vi "Runtime Test.vi"() -> ()   [LabVIEW 2015, in "Numeric Limit Compare Tests.lvlib"]
uses:
  Numeric Limit Compare Tests.lvlib
  Config/Numeric Limit Compare Config.lvclass
  <vilib>/NI/Tag Bus/tag/Data Type.ctl
  <vilib>/NI/Tag Bus Module Framework/channel/channel classification.ctl
  classes/Step/Execution/StepState.ctl
  classes/Step/Execution/Step State Enum.ctl
  classes/Step/Execution/Step Flow Control.ctl
  Config/Comparison Types.ctl
  Config/Numeric Limit Compare Config.lvclass/Numeric Limit Compare Config.ctl
  <vilib>/NI/Tag Bus/tag/tag descriptor.lvclass/tag descriptor.ctl
  <vilib>/NI/Tag Bus/table/data polymorphs/write one/write Double.vi
  <vilib>/NI/Tag Bus/table/data polymorphs/read one/read Boolean.vi
  Config/Write channel.vi
  Config/Write Comparison Type.vi
  Config/Write Lower Limit.vi
  Config/Write Negate Result.vi
  Config/Write Upper Limit_Limit.vi
  Config/Write Result Channel.vi
  <vilib>/NI/Tag Bus/tag/read tag name.vi
  <vilib>/NI/Tag Bus/tag/read data type.vi
  <vilib>/NI/Tag Bus/dictionary/locate tag.vi
  classes/Step/Execution/Step.lvclass
  <vilib>/NI/Tag Bus Module Framework/channel/TBM channel.lvclass
  <vilib>/NI/Tag Bus/tag/tag descriptor.lvclass
  <vilib>/NI/Tag Bus/dictionary/data dictionary.lvclass
  <vilib>/NI/Tag Bus/table/data table.lvlib
panel:
  out "result":bool
  in  "test value":dbl
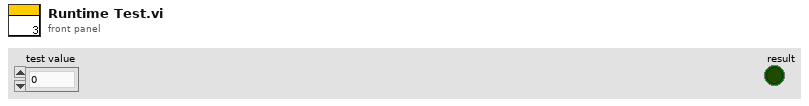
[diagram p1: front panel]
types:
  T1 = typedef "TBM channel.lvclass/channel classification.ctl" = enum16{"input data", "output data", "processing parameter", "processing result"}
  T2 = typedef "tag bus.lvlib/tag descriptor.lvclass/Data Type.ctl" = enum16{"Double", "Single", "I64", "I32", "I16", "I8", "U64", "U32", "U16", "U8", "Boolean", "String", "Array of Double", "Array of Single", "Array of I64", "Array of I32", "Array of I16", "Array of I8", "Array of U64", "Array of U32", "Array of U16", "Array of U8", "Array of Boolean", "Array of String"}
  T3 = typedef "Comparison Types.ctl" = enum16{"GELE (>=<=)", "GTLE(><=)", "GTLT(><)", "GELT(>=<)", "EQ(==)", "NE (!=)", "GT(>)", "LT(<)", "GE(>=)", "LE(<=)"}
  T4 = typedef "Step.lvclass/StepState.ctl" = cluster{"Step State":T5, "Flow Control":T6, "Jump Index":i32}
  T5 = typedef "Step.lvclass/Step State Enum.ctl" = enum16{"Start", "Skipped", "Timeout", "Completed", "Running", "Aborted"}
  T6 = typedef "Step.lvclass/Step Flow Control.ctl" = enum16{"Next Step", "Jump"}
  T7 = typedef "TBM channel.lvclass/data tables.ctl" = cluster{"input data":T8, "processing parameter":T8, "processing result":T8, "output data":T8}
  T8 = typedef "tag bus.lvlib/dictionary table pair.ctl" = cluster{"data dictionary":refnum<class "data dictionary.lvclass">, "data table":T9}
  T9 = typedef "tag bus.lvlib/data table.lvlib/data table.ctl" = cluster{"Double":dbl[], "Single":sgl[], "I64":i64[], "I32":i32[], "I16":i16[], "I8":i8[], "U64":u64[], "U32":u32[], "U16":u16[], "U8":u8[], "Boolean":bool[], "String":string[], "Array of Double":cluster{"DBL Array":dbl[]}[], "Array of Single":cluster{"SGL Array":sgl[]}[], "Array of I64":cluster{"I64 Array":i64[]}[], "Array of I32":cluster{"I32 Array":i32[]}[], "Array of I16":cluster{"I16 Array":i16[]}[], "Array of I8":cluster{"I8 Array":i8[]}[], "Array of U64":cluster{"U64 Array":u64[]}[], "Array of U32":cluster{"U32 Array":u32[]}[], "Array of U16":cluster{"U16 Array":u16[]}[], "Array of U8":cluster{"U8 Array":u8[]}[], "Array of Boolean":cluster{"Boolean Array":bool[]}[], "Array of String":cluster{"String Array":string[]}[]}
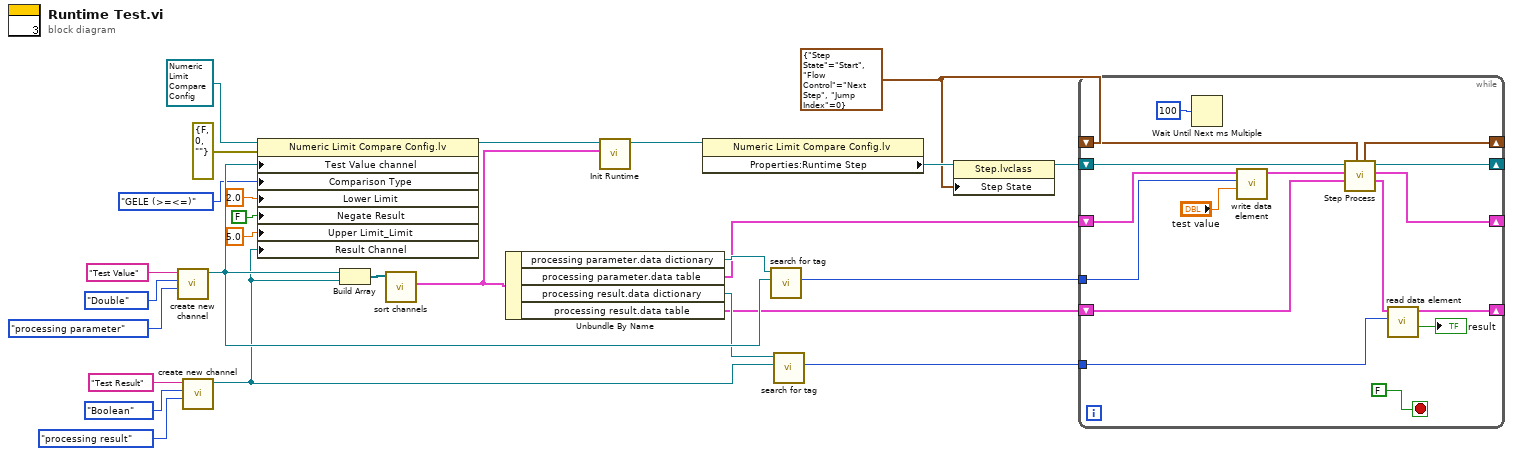
[diagram p0: block diagram]
diagram:
  w18 = T4 {"Step State"=enum."Start", "Flow Control"=enum."Next Step", "Jump Index"=0} ("Step State")
  n1 = call <vilib>:"create new channel.vi"("channel classification"=channel_classification."processing parameter", "data type"=Data_Type."Double", "channel name"="Test Value") -> ("channel"=w16:refnum<class "TBM channel.lvclass">)  [unwired: 8 in]
  n2 = call <vilib>:"create new channel.vi"("channel classification"=channel_classification."processing result", "data type"=Data_Type."Boolean", "channel name"="Test Result") -> ("channel"=w4:refnum<class "TBM channel.lvclass">)  [unwired: 8 in]
  n3 = property class="Numeric Limit Compare Config.lv"(reference=refnum<class "Numeric Limit Compare Config.lvclass"> refnum ("Numeric Limit Compare Config.lvclass"), error in=errorcluster {"status"=FALSE, "code"=0, "source"=""} ("error in (no error)"), "Test Value channel"=w16, "Comparison Type"=Comparison_Types."GELE (>=<=)", "Lower Limit"=2.0, "Negate Result"=FALSE, "Upper Limit_Limit"=5.0, "Result Channel"=w4) -> (reference out=w26:refnum<class "Numeric Limit Compare Config.lvclass">)  [unwired: 1 out]
  n4 = Build Array(w16, w4) -> (w22:refnum<class "TBM channel.lvclass">[])
  n5 = call <vilib>:"sort channels.vi"("channels in"=w22) -> ("data allocations"=w1:T7)  [unwired: 8 in, 2 out]
  n6 = Unbundle By Name(w1) -> ("processing parameter.data dictionary"=w17:refnum<class "data dictionary.lvclass">, "processing parameter.data table"=w15:T9, "processing result.data dictionary"=w5:refnum<class "data dictionary.lvclass">, "processing result.data table"=w3:T9)
  n7 = call-dynamic "Init Runtime.vi"("data allocations"=w1, "Numeric Limit Compare Config in"=w26) -> ("Numeric Limit Compare Config out"=w21:refnum<class "Numeric Limit Compare Config.lvclass">)  [unwired: 7 in, 2 out]
  n8 = property class="Numeric Limit Compare Config.lv"(reference=w21) -> ("Properties:Runtime Step"=w20:refnum<class "Step.lvclass">)  [unwired: 1 in, 2 out]
  n9 = call <vilib>:"search for tag.vi"("system tag"=w16, "data dictionary in"=w17) -> ("index"=w14:i32)  [unwired: 7 in, 2 out]
  n10 = call <vilib>:"search for tag.vi"("system tag"=w4, "data dictionary in"=w5) -> ("index"=w2:i32)  [unwired: 7 in, 2 out]
  n11 = property class="Step.lvclass"(reference=w20, "Step State"=w18) -> (reference out=w19:refnum<class "Step.lvclass">)  [unwired: 1 in, 1 out]
  n12 = while {
    shift-right: [w38] -> _
    shift-left: w19 -> [w43]
    shift-right: [w39] -> _
    shift-left: w18 -> [w40]
    shift-right: [w35] -> _
    shift-left: w15 -> [w37]
    tunnel: w14 -> [w34]
    tunnel: w2 -> [w33]
    shift-right: [w31] -> _
    shift-left: w3 -> [w29]
    stop <- FALSE ("stop") stop-if-true
    n13 = Wait Until Next ms Multiple(millisecond multiple=u32 100) -> ()  [unwired: 1 out]
    n14 = call-poly <vilib>:"write data element.vi"("value"="test value", "index"=w34, "data table in"=w37) -> ("data table out"=w36:T9)  [unwired: 8 in]
    n15 = call-dynamic "Step Process.vi"("Step State in"=w40, "result allocation"=w29, "parameters"=w36, "Step in"=w43) -> ("results"=w28:T9, "parameter allocation"=w35:T9, "Step out"=w38:refnum<class "Step.lvclass">, "Step State out"=w39:T4)  [unwired: 3 in, 1 out]
    n16 = call-poly <vilib>:"read data element.vi"("index"=w33, "data table in"=w28) -> ("value"=→"result":bool, "data table out"=w31:T9)  [unwired: 8 in]
  }
